vi "Write ModeArray.vi"(8 "error in (no error)":errorcluster, 10 "ModeArray":T1(array[cluster])=[{"Mode"="Continue", "ModeTag"="MODE_CONTINUE", "Disables?"=TRUE}, {"Mode"="Ramp", "ModeTag"="MODE_RAMP", "Disables?"=FALSE}, {"Mode"="Loop", "ModeTag"="MODE_LOOP", "Disables?"=TRUE}, {"Mode"="EndLoop", "ModeTag"="MODE_ENDLOOP", "Disables?"=TRUE}], 11 "ModeCol in":refnum<class "ModeCol.lvclass">) -> (0 "error out":errorcluster, 3 "ModeCol out":refnum<class "ModeCol.lvclass">)   [LabVIEW 2013, in "ModeCol.lvclass"]
uses:
  ModeCol.lvclass
  ModeCol.lvclass/ModeCol.ctl
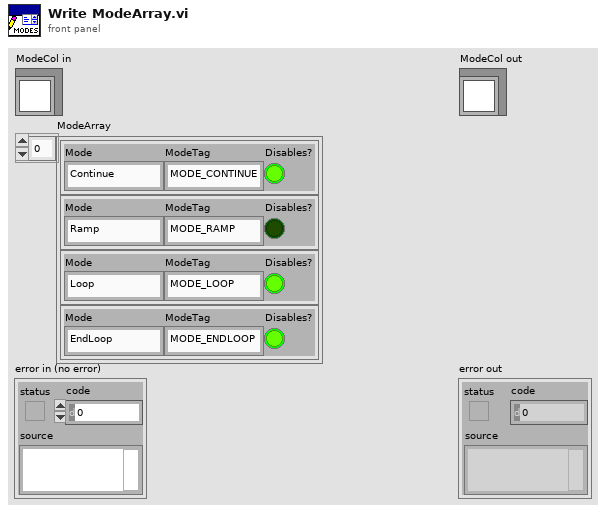
[diagram p1: front panel]
types:
  T1 = cluster{"Mode":string, "ModeTag":string, "Disables?":bool}[]
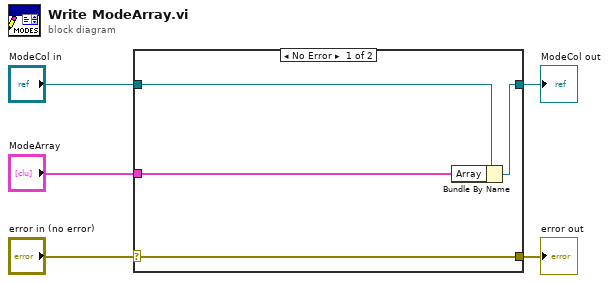
[diagram p0: block diagram]
diagram:
  n1 = case shown="No Error" "error in (no error)" {
    selector: "error in (no error)" -> [w9 w10]
    tunnel: [w9 w10] -> w4
    tunnel: [w7 w11] -> w2
    tunnel: "ModeCol in" -> [w8 w11]
    tunnel: "ModeArray" -> [w6 _]
    frame No Error {
      n2 = Bundle By Name(cluster=w8, "Array"=w6) -> (w7:refnum<class "ModeCol.lvclass">)
    }
    frame Error {
    }
  }
  "error out" <- w4
  "ModeCol out" <- w2
